vi "A - write log line.vi"(8 "error in":errorcluster, 9 "temperature boxes":T1={"LTC21 Address"="GPIB0::15::INSTR", "ITC503 Address"="GPIB0::24::INSTR", "ITC temperature"=299.2, "ITC set temperature"=295.0, "LTC temperature"=0.0, "heater"=0.0, "gas flow"=90.0, "P"=10.0, "D"=1.0, "I"=3.0, "ITC state"="X0A1C2S00H1L0\r", "nonzero temperature"=0.0, "Magn Field (T)"=0.0, "LakeShore340"="", "LS340 Adress"=0, "Sample Temperature Source"=enum."read T <- LakeShore 340", "Neocera sensor"=1}, 10 "Basename":string="Control_ITC_Log_", 11 "Base Path":path) -> (0 "error out":errorcluster, 3 "saving log to":string="C:\\data\\RUS\\Experiment\\YBCO_4\\Sweep10\\Control_ITC_Log_061411.dat")   [LabVIEW 2012]
uses:
  state.ctl
  Sample_Temperature_Source_Control.ctl
  <vilib>/Utility/file.llb/Write To Spreadsheet File (string).vi
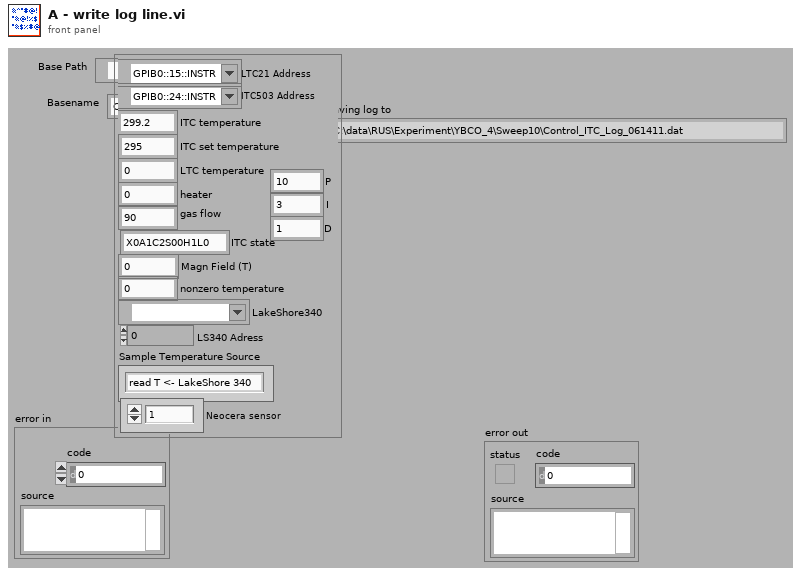
[diagram p1: front panel]
types:
  T1 = typedef "state.ctl" = cluster{"LTC21 Address":refnum<visa-resource-name>, "ITC503 Address":refnum<visa-resource-name>, "ITC temperature":dbl, "ITC set temperature":dbl, "LTC temperature":dbl, "heater":dbl, "gas flow":dbl, "P":dbl, "D":dbl, "I":dbl, "ITC state":string, "nonzero temperature":dbl, "Magn Field (T)":dbl, "LakeShore340":refnum<visa-resource-name>, "LS340 Adress":i16, "Sample Temperature Source":T2, "Neocera sensor":i32}
  T2 = typedef "Sample_Temperature_Source_Control.ctl" = enum16{"read T <- LakeShore 340", "read T <- Neocera"}
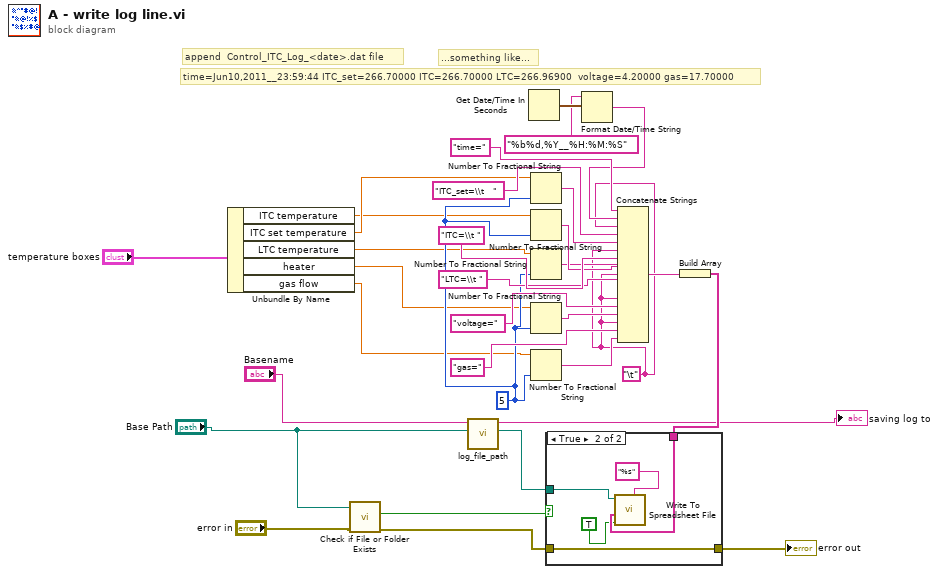
[diagram p0: block diagram]
diagram:
  w16 = "\t"
  w15 = i16 5 ("width (-)")
  # "...something like..."
  # "time=Jun10,2011__23:59:44\tITC_set=266.70000\tITC=266.70000\tLTC=266.96900\t\tvoltage=4.20000\tgas=17.70000"
  # "append  Control_ITC_Log_<date>.dat file"
  n1 = Unbundle By Name("temperature boxes") -> ("ITC temperature"=w13:dbl, "ITC set temperature"=w14:dbl, "LTC temperature"=w12:dbl, "heater"=w11:dbl, "gas flow"=w10:dbl)
  n2 = call <vilib>:"Check if File or Folder Exists.vi"("error in (no error)"="error in", "path"="Base Path") -> ("error out"=w2:errorcluster, "file or folder exists?"=w4:bool)  [unwired: 7 in, 1 out]
  n3 = call "log_file_path.vi"("base path in"="Base Path", "base name in"="Basename") -> ("path out"=w8:path, "string path out"=→"saving log to":string)  [unwired: 8 in]
  n4 = Get Date/Time In Seconds() -> (seconds since 1Jan1904=w32:timestamp)
  n5 = Number To Fractional String(number=w14, precision (6)=w15) -> (F-format string=w27:string)  [unwired: 2 in]
  n6 = Number To Fractional String(number=w13, precision (6)=w15) -> (F-format string=w25:string)  [unwired: 2 in]
  n7 = Number To Fractional String(number=w12, precision (6)=w15) -> (F-format string=w23:string)  [unwired: 2 in]
  n8 = Number To Fractional String(number=w11, precision (6)=w15) -> (F-format string=w19:string)  [unwired: 2 in]
  n9 = Number To Fractional String(number=w10, precision (6)=w15) -> (F-format string=w17:string)  [unwired: 2 in]
  n10 = Format Date/Time String(time format string (%c)="%b%d,%Y__%H:%M:%S", seconds (now)=w32) -> (date/time string=w30:string)  [unwired: 1 in]
  n11 = Concatenate Strings("time=" ("string"), w30, w16, "ITC_set=\\t   " ("string"), w27, w16, "ITC=\\t " ("string"), w25, w16, "LTC=\\t " ("string"), w23, w16, "voltage=" ("string"), w19, w16, "gas=" ("string"), w17) -> (w22:string)
  n12 = Build Array(w22) -> (w21:string[])
  n13 = case shown="True" w4 {
    tunnel: w21 -> [_ w38]
    tunnel: w8 -> [_ w37]
    tunnel: [w33 w34] -> w3
    tunnel: w2 -> [w33 w34]
    frame False {
    }
    frame True {
      n14 = call-poly <vilib>:"Write To Spreadsheet File.vi"("format (%s)"="%s", "append to file? (new file:F)"=TRUE, "1D data"=w38, "file path (dialog if empty)"=w37) -> ()  [unwired: 4 in, 1 out]
    }
  }
  "error out" <- w3
